vi "New Panel Controller.vi"(0 "reference in":refnum<class "Panel Controller.lvclass">, 5 "error in (no error)":errorcluster) -> (14 "reference out":refnum<class "Panel Controller.lvclass">, 19 "error out":errorcluster)   [LabVIEW 2015, in "Panel Controller.lvclass"]
uses:
  Panel Controller.lvclass
  Panel GUI Manager/Panel GUI Manager.lvclass
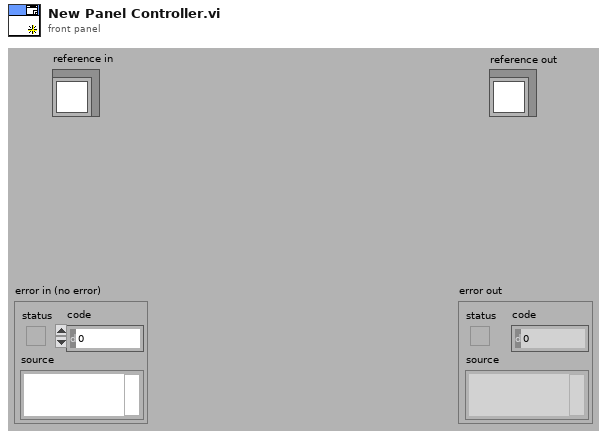
[diagram p1: front panel]
types:
  T1 = typedef "Panel Controller.lvclass/ObjectAttributes.ctl" = cluster{"Sub Panel Ref":refnum<vi>, "Panel_Q":refnum<queue>, "VI Running Refnum":refnum<vi>, "Brower Controller_Q":refnum<class "Message Enqueuer.lvclass">, "GUI Control Builder Director.lvclass":refnum<class "GUI Control Builder Director.lvclass">, "Panel GUI Manager.lvclass":refnum<class "Panel GUI Manager.lvclass">}
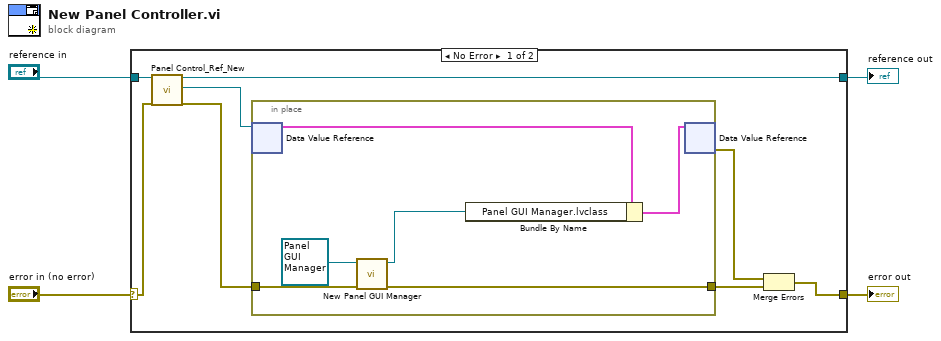
[diagram p0: block diagram]
diagram:
  n1 = case shown="No Error" "error in (no error)" {
    selector: "error in (no error)" -> [w11 w20]
    tunnel: [w8 w20] -> w3
    tunnel: "reference in" -> [w12 w19]
    tunnel: [w10 w19] -> w1
    frame No Error {
      n2 = call "Panel Control_Ref_New.vi"("reference in"=w12, "error in (no error)"=w11) -> ("reference out"=w10:refnum<class "Panel Controller.lvclass">, "DVRRefOut"=w7:refnum<data-value>, "error out"=w6:errorcluster)  [unwired: 14 in, 1 out]
      n3 = in-place {
        in-place-border: w6 -> [w15]
        in-place-border: [w14] -> w5
        n4 = in-place-dvr #1(w7) -> (w18:T1)  [unwired: 1 out]
        n5 = call "New Panel GUI Manager.vi"("error in (no error)"=w15, "Panel GUI Manager in"=refnum<class "Panel GUI Manager.lvclass"> refnum ("Panel GUI Manager.lvclass")) -> ("error out"=w14:errorcluster, "Panel GUI Manager out"=w16:refnum<class "Panel GUI Manager.lvclass">)  [unwired: 8 in]
        n6 = Bundle By Name(cluster=w18, "Panel GUI Manager.lvclass"=w16) -> (w13:T1)
        n7 = in-place-dvr #1(w13) -> (w9:errorcluster)  [unwired: 1 out]
      }
      n8 = Merge Errors(w9, w5) -> (w8:errorcluster)
    }
    frame Error {
    }
  }
  "error out" <- w3
  "reference out" <- w1
